vi "Pump Status.vi"(8 "error in (no error)":errorcluster, 11 "Pump Calibration Config in":T1={"Settings"={"Cycle Period"=500.0, "Ismatech"={"VISA resource name"="", "Simulated?"=TRUE, "Pump Number"=1.0, "Reverse?"=FALSE}, "Masterflex"={"VISA resource name"="", "Simulated?"=TRUE, "Pump Number"=1.0, "Reverse?"=FALSE}, "Bronkhorst M13 Flow Meter"={"VISA resource name"="", "Simulated?"=TRUE}, "PID 2 Parameters"={"Input Device"=enum."Default", "Output Device"=enum."Default"}, "Bronkhorst M14"={"VISA resource name"="", "Simulated?"=FALSE}, "Tacmina Settings"={"Analog DAQ Task"="", "Digital DAQ Task"=""}, "KNF SIMDOS Settings"={"VISA resource name"="", "Simulated?"=TRUE}, "VICI M50 Settings"={"VISA resource name"="", "Simulated?"=TRUE, "Pump Letter"="", "Reverse?"=FALSE}, "FLOM Settings"={"VISA resource name"="", "Simulated?"=TRUE, "Pump Number"=0.0}, "Calibration Limits"={"Minimum (ml/min)"=0.0, "Maximum (ml/min)"=0.0, "Steps"=0.0}, "SSI PR Settings"={"VISA resource name"="", "Simulated?"=FALSE}}, "Flowmeter Output"=0.0, "Density"=0.0, "FL Temp"=0.0, "Speed %"=0.0, "File Refnum"=refnum, "Pump On?"=enum."Not Initialized"} {"Settings"."Masterflex"."Pump Number" min=1.0 max=20.0 step=1.0; "Settings"."Ismatech"."Pump Number" min=1.0 max=20.0 step=1.0}) -> (0 "error out":errorcluster, 3 "Pump Calibration Config out":T1={"Settings"={"Cycle Period"=500.0, "Ismatech"={"VISA resource name"="", "Simulated?"=TRUE, "Pump Number"=1.0, "Reverse?"=FALSE}, "Masterflex"={"VISA resource name"="", "Simulated?"=TRUE, "Pump Number"=1.0, "Reverse?"=FALSE}, "Bronkhorst M13 Flow Meter"={"VISA resource name"="", "Simulated?"=TRUE}, "PID 2 Parameters"={"Input Device"=enum."Default", "Output Device"=enum."Default"}, "Bronkhorst M14"={"VISA resource name"="", "Simulated?"=FALSE}, "Tacmina Settings"={"Analog DAQ Task"="", "Digital DAQ Task"=""}, "KNF SIMDOS Settings"={"VISA resource name"="", "Simulated?"=TRUE}, "VICI M50 Settings"={"VISA resource name"="", "Simulated?"=TRUE, "Pump Letter"="", "Reverse?"=FALSE}, "FLOM Settings"={"VISA resource name"="", "Simulated?"=TRUE, "Pump Number"=0.0}, "Calibration Limits"={"Minimum (ml/min)"=0.0, "Maximum (ml/min)"=0.0, "Steps"=0.0}, "SSI PR Settings"={"VISA resource name"="", "Simulated?"=FALSE}}, "Flowmeter Output"=0.0, "Density"=0.0, "FL Temp"=0.0, "Speed %"=0.0, "File Refnum"=refnum, "Pump On?"=enum."Not Initialized"} {"Settings"."Masterflex"."Pump Number" min=1.0 max=20.0 step=1.0; "Settings"."Ismatech"."Pump Number" min=1.0 max=20.0 step=1.0})   [LabVIEW 2018, in "Calibration.lvlib" / "Engine.lvlib"]
uses:
  Engine.lvlib
  Pump Calibration Config.ctl
  Pfizer Timed Seq/Software/Ismatec ISM 831C/Controls/Ismatech Settings Cluster.ctl
  Pfizer Timed Seq/Software/Masterflex 7550-30/Controls/Settings Cluster.ctl
  Pfizer Timed Seq/Software/Bronkhorst M13 Flow Meter/Settings Cluster.ctl
  Pfizer Timed Seq/Software/Measure Instrument/PID Input Enum.ctl
  Pfizer Timed Seq/Software/Measure Instrument/PID 2 Output Enum.ctl
  Pfizer Timed Seq/Software/Mettler Toledo/Controls/Settings Cluster.ctl
  Pfizer Timed Seq/Software/Tacmina QI/Tacmina QI DAQ Setting.ctl
  Pfizer Timed Seq/Software/KNF Pump/Settings Cluster plus SIMDOS.ctl
  Pfizer Timed Seq/Software/VICI M50 Party Mode/Settings Cluster.ctl
  Pfizer Timed Seq/Software/FLOM Pump/Settings Cluster.ctl
  Pfizer Timed Seq/Software/SSI PR Class/SSI PR Settings Cluster.ctl
  Pfizer Timed Seq/Software/Ismatec ISM 831C/Ismatec ISM 831C.lvlib
  Pfizer Timed Seq/Software/Masterflex 7550-30/Masterflex 7550-30.lvlib
  Pfizer Timed Seq/Software/VICI M50 Party Mode/VICI M50 Party Mode.lvlib
  Pfizer Timed Seq/Software/Tacmina QI/Tacmina QI.lvlib
  Pfizer Timed Seq/Software/KNF Pump/KNF SIMDOS.lvlib
  Pfizer Timed Seq/Software/FLOM Pump/FLOM Pump.lvlib
  Pfizer Timed Seq/Software/SSI PR Class/SSI PR Pump.lvlib
  Pfizer Timed Seq/Software/Bronkhorst M13 Flow Meter/Bronkhorst M13 Flow Meter.lvlib
  Pfizer Timed Seq/Software/Mettler Toledo/Mettler Toledo.lvlib
  Pfizer Timed Seq/Software/Calibration VIs/Calibration.lvlib
panel:
  # "Output Instruments"
  # "Input Instruments"
  # "Output Instruments"
  # "Input Instruments"
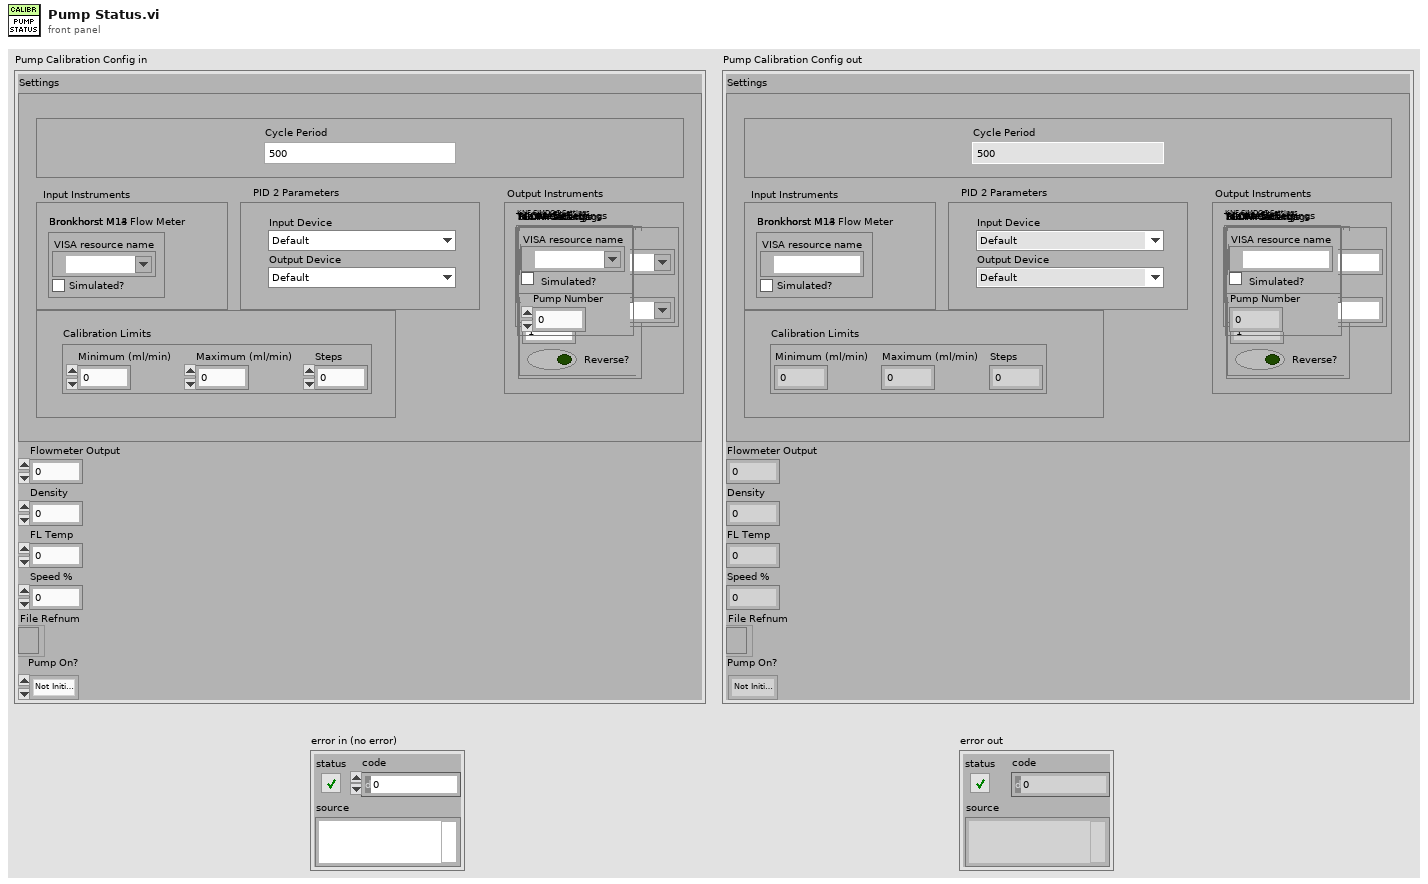
[diagram p1: front panel]
types:
  T1 = typedef "Calibration.lvlib/Pump Calibration Config.ctl" = cluster{"Settings":cluster{"Cycle Period":dbl, "Ismatech":T2, "Masterflex":T3, "Bronkhorst M13 Flow Meter":T4, "PID 2 Parameters":cluster{"Input Device":T5, "Output Device":T6}, "Bronkhorst M14":T7, "Tacmina Settings":T8, "KNF SIMDOS Settings":T9, "VICI M50 Settings":T10, "FLOM Settings":T11, "Calibration Limits":cluster{"Minimum (ml/min)":dbl, "Maximum (ml/min)":dbl, "Steps":dbl}, "SSI PR Settings":T12}, "Flowmeter Output":dbl, "Density":dbl, "FL Temp":dbl, "Speed %":dbl, "File Refnum":refnum<file>, "Pump On?":enum16{"Off", "On", "Not Initialized"}}
  T2 = typedef "Ismatec ISM 831C.lvlib/Ismatech Settings Cluster.ctl" = cluster{"VISA resource name":refnum<visa-resource-name>, "Simulated?":bool, "Pump Number":dbl, "Reverse?":bool}
  T3 = typedef "Masterflex 7550-30.lvlib/Settings Cluster.ctl" = cluster{"VISA resource name":refnum<visa-resource-name>, "Simulated?":bool, "Pump Number":dbl, "Reverse?":bool}
  T4 = typedef "Bronkhorst M13 Flow Meter.lvlib/Settings Cluster.ctl" = cluster{"VISA resource name":refnum<visa-resource-name>, "Simulated?":bool}
  T5 = typedef "PID Input Enum.ctl" = enum16{"Default", "Bronkhorst M13", "Bronkhorst M14", "Scale Rate of Change"}
  T6 = typedef "PID 2 Output Enum.ctl" = enum16{"Default", "Ismatec ISM 831C", "Masterflex 7550-30", "VICI", "Tacmina QI", "KNF SIMDOS", "ASIA Type C", "FLOM UI-22-11", "SSI PR"}
  T7 = typedef "Mettler Toledo.lvlib/Settings Cluster.ctl" = cluster{"VISA resource name":refnum<visa-resource-name>, "Simulated?":bool}
  T8 = typedef "Tacmina QI.lvlib/Tacmina QI DAQ Setting.ctl" = cluster{"Analog DAQ Task":refnum<k21>, "Digital DAQ Task":refnum<k21>}
  T9 = typedef "KNF SIMDOS.lvlib/Settings Cluster plus SIMDOS.ctl" = cluster{"VISA resource name":refnum<visa-resource-name>, "Simulated?":bool}
  T10 = typedef "VICI M50 Party Mode.lvlib/Settings Cluster.ctl" = cluster{"VISA resource name":refnum<visa-resource-name>, "Simulated?":bool, "Pump Letter":string, "Reverse?":bool}
  T11 = typedef "FLOM Pump.lvlib/Settings Cluster.ctl" = cluster{"VISA resource name":refnum<visa-resource-name>, "Simulated?":bool, "Pump Number":dbl}
  T12 = typedef "SSI PR Pump.lvlib/SSI PR Settings Cluster.ctl" = cluster{"VISA resource name":refnum<visa-resource-name>, "Simulated?":bool}
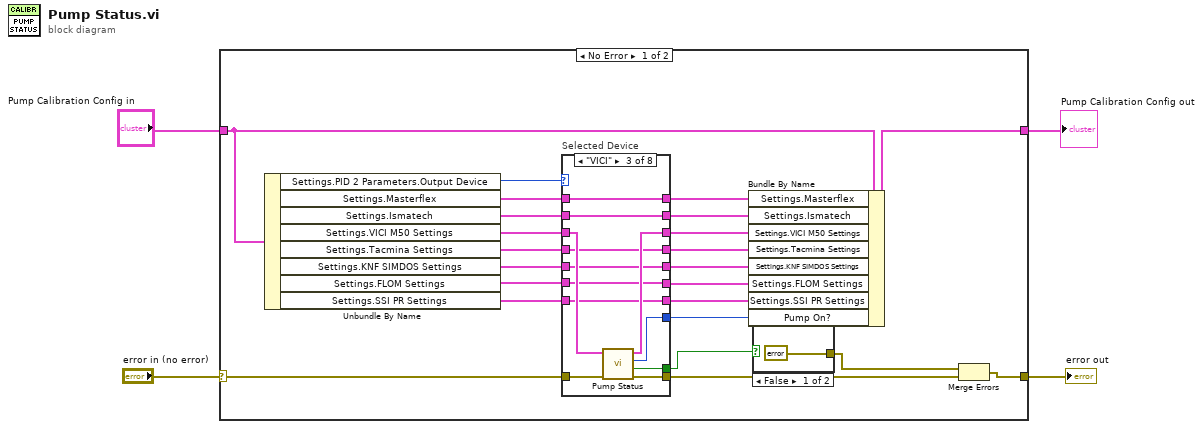
[diagram p0: block diagram]
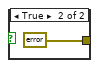
[diagram p2: hidden frame]
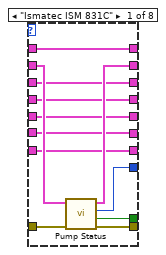
[diagram p3: hidden frame]
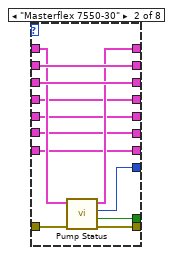
[diagram p4: hidden frame]
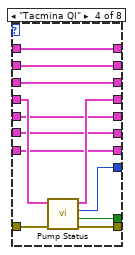
[diagram p5: hidden frame]
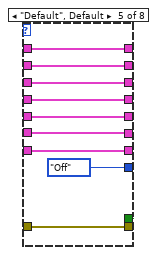
[diagram p6: hidden frame]
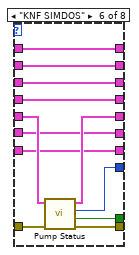
[diagram p7: hidden frame]
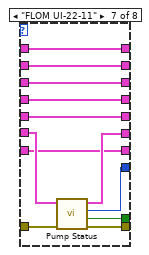
[diagram p8: hidden frame]
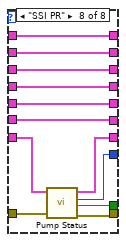
[diagram p9: hidden frame]
diagram:
  n1 = case shown="No Error" "error in (no error)" {
    selector: "error in (no error)" -> [w19 w125]
    tunnel: [w10 w125] -> w3
    tunnel: "Pump Calibration Config in" -> [w22 w124]
    tunnel: [w27 w124] -> w1
    frame No Error {
      n2 = Unbundle By Name(w22) -> ("Settings.PID 2 Parameters.Output Device"=w12:T6, "Settings.Masterflex"=w26:T3, "Settings.Ismatech"=w25:T2, "Settings.VICI M50 Settings"=w24:T10, "Settings.Tacmina Settings"=w21:T8, "Settings.KNF SIMDOS Settings"=w20:T9, "Settings.FLOM Settings"=w23:T11, "Settings.SSI PR Settings"=w7:T12)
      n3 = case "Selected Device" shown="\"VICI\"" w12 {
        tunnel: w26 -> [w41 w49 w64 w77 w87 w99 w111 w112]
        tunnel: [w41 w50 w64 w77 w87 w99 w111 w112] -> w18
        tunnel: w25 -> [w39 w53 w65 w76 w86 w98 w110 w123]
        tunnel: [w40 w51 w61 w73 w80 w95 w106 w117] -> w8
        tunnel: w19 -> [w31 w43 w55 w67 w80 w89 w101 w118]
        tunnel: [w38 w53 w65 w76 w86 w98 w110 w123] -> w17
        tunnel: w24 -> [w36 w52 w62 w75 w85 w97 w109 w122]
        tunnel: [w36 w52 w63 w75 w85 w97 w109 w122] -> w16
        tunnel: w21 -> [w37 w48 w60 w74 w84 w96 w108 w121]
        tunnel: [w37 w48 w60 w72 w84 w96 w108 w121] -> w15
        tunnel: [w35 w47 w59 w71 w83 w94 w107 w120] -> w14
        tunnel: w20 -> [w35 w47 w59 w71 w83 w93 w107 w120]
        tunnel: [w34 w46 w58 w70 enum16{"Off", "On", "Not Initialized"}."Off" ("Pump On?") w92 w103 w115] -> w6
        tunnel: [w33 w45 w57 w69 w81 w91 w105 w119] -> w13
        tunnel: w23 -> [w33 w45 w57 w69 w81 w91 w104 w119]
        tunnel: [w32 w44 w56 w68 FALSE ("Connection Error") w90 w102 w116] -> w11
        tunnel: w7 -> [w30 w42 w54 w66 w78 w88 w100 w114]
        tunnel: [w30 w42 w54 w66 w78 w88 w100 w113] -> w5
        frame "Ismatec ISM 831C" {
          n4 = call "Pump Status.vi"("error in (no error)"=w31, "Ismatech Settings"=w39) -> ("error out"=w40:errorcluster, "Connection Error"=w32:bool, "Pump On?"=w34:enum16{"Off", "On", "Not Initialized"}, "Ismatech Settings"=w38:T2)  [unwired: 6 in]
        }
        frame "Masterflex 7550-30" {
          n5 = call "Pump Status.vi"("error in (no error)"=w43, "Masterflex Settings in"=w49) -> ("error out"=w51:errorcluster, "Connection Error"=w44:bool, "Pump On?"=w46:enum16{"Off", "On", "Not Initialized"}, "Masterflex Settings out"=w50:T3)  [unwired: 6 in]
        }
        frame "VICI" {
          n6 = call "Pump Status.vi"("error in (no error)"=w55, "VICI Settings"=w62) -> ("error out"=w61:errorcluster, "Connection Error"=w56:bool, "Pump On?"=w58:enum16{"Off", "On", "Not Initialized"}, "VICI Settings"=w63:T10)  [unwired: 6 in]
        }
        frame "Tacmina QI" {
          n7 = call "Pump Status.vi"("error in"=w67, "Tacmina Settings in"=w74) -> ("error out"=w73:errorcluster, "Connection Error"=w68:bool, "Pump On?"=w70:enum16{"Off", "On", "Not Initialized"}, "Tacmina Settings out"=w72:T8)  [unwired: 6 in]
        }
        frame "Default", Default {
        }
        frame "KNF SIMDOS" {
          n8 = call "Pump Status.vi"("error in (no error)"=w89, "KNF Settings"=w93) -> ("error out"=w95:errorcluster, "Connection Error"=w90:bool, "Pump On?"=w92:enum16{"Off", "On", "Not Initialized"}, "KNF Settings"=w94:T9)  [unwired: 6 in]
        }
        frame "FLOM UI-22-11" {
          n9 = call "Pump Status.vi"("error in (no error)"=w101, "FLOM Settings In"=w104) -> ("error out"=w106:errorcluster, "Connection Error"=w102:bool, "Pump On?"=w103:enum16{"Off", "On", "Not Initialized"}, "FLOM Settings Out"=w105:T11)  [unwired: 4 in, 2 out]
        }
        frame "SSI PR" {
          n10 = call "Pump Status.vi"("error in (no error)"=w118, "SSI PR Settings"=w114) -> ("error out"=w117:errorcluster, "Connection Error"=w116:bool, "Pump On?"=w115:enum16{"Off", "On", "Not Initialized"}, "SSI PR Settings"=w113:T12)  [unwired: 4 in, 2 out]
        }
      }
      n11 = Bundle By Name(cluster=w22, "Settings.Masterflex"=w18, "Settings.Ismatech"=w17, "Settings.VICI M50 Settings"=w16, "Settings.Tacmina Settings"=w15, "Settings.KNF SIMDOS Settings"=w14, "Settings.FLOM Settings"=w13, "Settings.SSI PR Settings"=w5, "Pump On?"=w6) -> (w27:T1)
      n12 = case shown="False" w11 {
        tunnel: [errorcluster {"status"=FALSE, "code"=0, "source"=""} ("error constant") errorcluster {"status"=TRUE, "code"=3, "source"="Pump Connection Error"} ("error constant")] -> w9
        frame False {
        }
        frame True {
        }
      }
      n13 = Merge Errors(w9, w8) -> (w10:errorcluster)
    }
    frame Error {
    }
  }
  "error out" <- w3
  "Pump Calibration Config out" <- w1
